vi "to DBL.vi"(8 "error in (no error)":errorcluster, 11 "MessagePackNumeric in":refnum<class "MessagePackNumeric.lvclass">) -> (0 "error out":errorcluster, 2 "Numeric":dbl, 3 "MessagePackNumeric out":refnum<class "MessagePackNumeric.lvclass">)   [LabVIEW 2020, in "MessagePack.lvlib" / "MessagePackNumeric.lvclass"]
uses:
  MessagePackNumeric.lvclass
  MessagePackNumeric.lvclass/MessagePackNumeric.ctl
  <vilib>/Utility/error.llb/Error Cluster From Error Code.vi
  <vilib>/ErrorRing/Error Ring.xnode
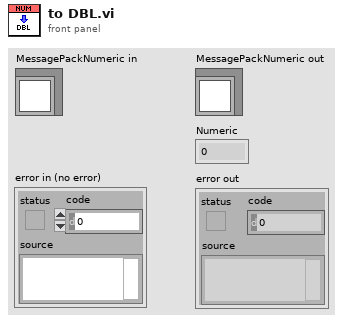
[diagram p1: front panel]
types:
  T1 = typedef "MessagePack.lvlib/MsgPack Object Types.ctl" = enum16{"UNSUPPORTED", "POSINT", "NEGINT", "FIXMAP", "FIXARRAY", "FIXSTR", "NIL", "FALSE", "TRUE", "BIN8", "BIN16", "BIN32", "EXT8", "EXT16", "EXT32", "FLOAT32", "FLOAT64", "UINT8", "UINT16", "UINT32", "UINT64", "INT8", "INT16", "INT32", "INT64", "FIXEXT1", "FIXEXT2", "FIXEXT4", "FIXEXT8", "FIXEXT16", "STR8", "STR16", "STR32", "ARRAY16", "ARRAY32", "MAP16", "MAP32"}
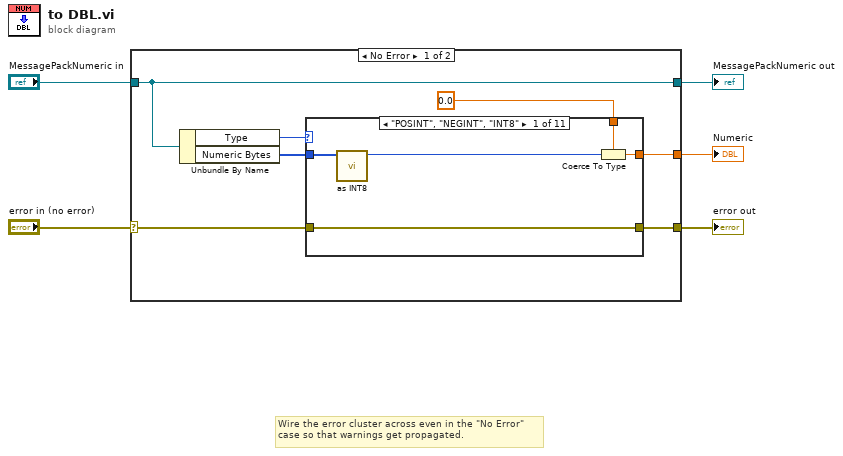
[diagram p0: block diagram]
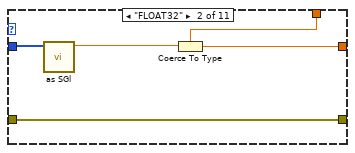
[diagram p2: hidden frame]
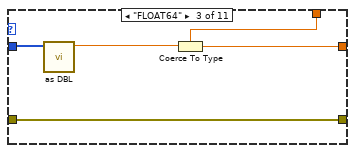
[diagram p3: hidden frame]
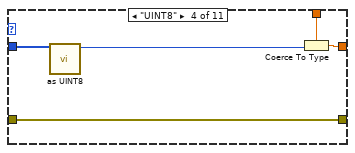
[diagram p4: hidden frame]
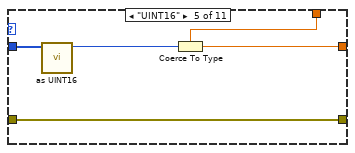
[diagram p5: hidden frame]
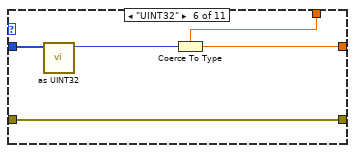
[diagram p6: hidden frame]
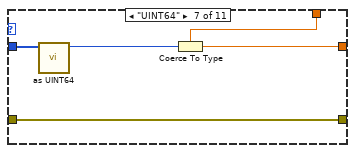
[diagram p7: hidden frame]
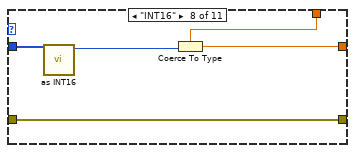
[diagram p8: hidden frame]
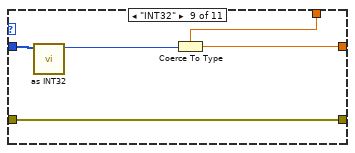
[diagram p9: hidden frame]
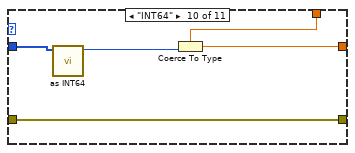
[diagram p10: hidden frame]
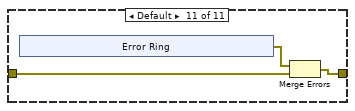
[diagram p11: hidden frame]
diagram:
  # "Wire the error cluster across even in the \"No Error\"\ncase so that warnings get propagated."
  n1 = case shown="No Error" "error in (no error)" {
    selector: "error in (no error)" -> [w7 w71]
    tunnel: [w6 w71] -> w4
    tunnel: [w12 w70] -> w2
    tunnel: "MessagePackNumeric in" -> [w12 w70]
    tunnel: [w9 _] -> w1
    frame No Error {
      n2 = Unbundle By Name(w12) -> ("Type"=w11:T1, "Numeric Bytes"=w10:u8[])
      n3 = case shown="\"POSINT\", \"NEGINT\", \"INT8\"" w11 {
        tunnel: w10 -> [w17 w19 w24 w30 w35 w40 w45 w50 w55 w60 _]
        tunnel: [w16 w22 w27 w32 w37 w42 w47 w52 w57 w62 _] -> w9
        tunnel: 0.0 ("type") -> [w15 w21 w26 w31 w36 w41 w46 w51 w56 w61 _]
        tunnel: w7 -> [w13 w18 w23 w28 w33 w38 w43 w48 w53 w58 w64]
        tunnel: [w13 w18 w23 w28 w33 w38 w43 w48 w53 w58 w63] -> w6
        frame "POSINT", "NEGINT", "INT8" {
          n4 = call "as INT8.vi"("bytes"=w17) -> ("INT8"=w14:i8)  [unwired: 10 in]
          n5 = Coerce To Type(0:w14, 1:w15) -> (2:w16:dbl)
        }
        frame "FLOAT32" {
          n6 = call "as SGl.vi"("bytes"=w19) -> ("SGL"=w20:sgl)  [unwired: 10 in]
          n7 = Coerce To Type(0:w20, 1:w21) -> (2:w22:dbl)
        }
        frame "FLOAT64" {
          n8 = call "as DBL.vi"("bytes"=w24) -> ("DBL"=w25:dbl)  [unwired: 10 in]
          n9 = Coerce To Type(0:w25, 1:w26) -> (2:w27:dbl)
        }
        frame "UINT8" {
          n10 = call "as UINT8.vi"("bytes"=w30) -> ("UINT8"=w29:u8)  [unwired: 10 in]
          n11 = Coerce To Type(0:w29, 1:w31) -> (2:w32:dbl)
        }
        frame "UINT16" {
          n12 = call "as UINT16.vi"("bytes"=w35) -> ("UINT16"=w34:u16)  [unwired: 10 in]
          n13 = Coerce To Type(0:w34, 1:w36) -> (2:w37:dbl)
        }
        frame "UINT32" {
          n14 = call "as UINT32.vi"("bytes"=w40) -> ("UINT32"=w39:u32)  [unwired: 10 in]
          n15 = Coerce To Type(0:w39, 1:w41) -> (2:w42:dbl)
        }
        frame "UINT64" {
          n16 = call "as UINT64.vi"("bytes"=w45) -> ("UINT64"=w44:u64)  [unwired: 10 in]
          n17 = Coerce To Type(0:w44, 1:w46) -> (2:w47:dbl)
        }
        frame "INT16" {
          n18 = call "as INT16.vi"("bytes"=w50) -> ("INT8"=w49:i16)  [unwired: 10 in]
          n19 = Coerce To Type(0:w49, 1:w51) -> (2:w52:dbl)
        }
        frame "INT32" {
          n20 = call "as INT32.vi"("bytes"=w55) -> ("INT32"=w54:i32)  [unwired: 10 in]
          n21 = Coerce To Type(0:w54, 1:w56) -> (2:w57:dbl)
        }
        frame "INT64" {
          n22 = call "as INT64.vi"("bytes"=w60) -> ("INT64"=w59:i64)  [unwired: 10 in]
          n23 = Coerce To Type(0:w59, 1:w61) -> (2:w62:dbl)
        }
        frame Default {
          n24 = xnode "Error Ring"() -> ("error out"=w65:errorcluster)
          n25 = Merge Errors(w65, w64) -> (w63:errorcluster)
        }
      }
    }
    frame Error {
    }
  }
  "error out" <- w4
  "MessagePackNumeric out" <- w2
  "Numeric" <- w1
